vi "mapRotAngleByTiltXY.vi"(8 "error in (no error)":errorcluster, 9 "Tilt Angle (degree)":cluster{"Tile X":dbl, "Tilt Y":dbl}, 10 "Rotation Angle in Deg":dbl, 11 "CamRot in":refnum<class "CamRot.lvclass">) -> (0 "error out":errorcluster, 2 "Mapped Rotation Angle in Deg":dbl, 3 "CamRot out":refnum<class "CamRot.lvclass">)   [LabVIEW 2016, in "OfcFunc.lvlib" / "CamRot.lvclass"]
doc: "Map the rotation angle by tilt x, y axis. The input rotation angle (theta') is defined on x', y'-plane, which is tilted from x, y-plane. The output rotation angle (theta) is defined on x, y-plane. The tilt angles in inputs are defined as tilt x'-x and tilt y'-y."
uses:
  CamRot.lvclass
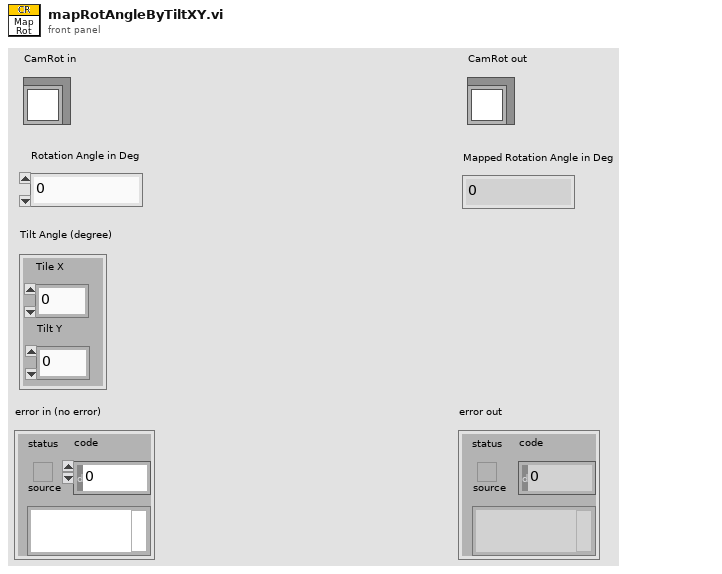
[diagram p1: front panel]
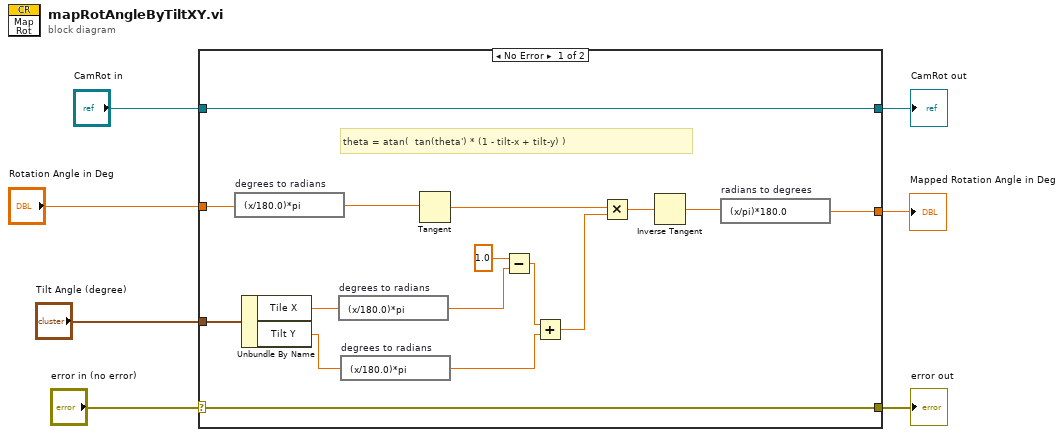
[diagram p0: block diagram]
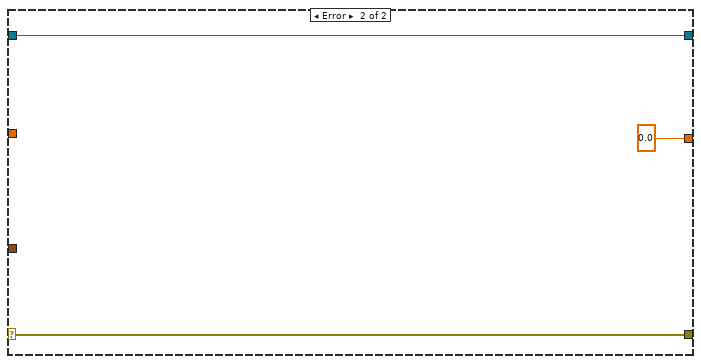
[diagram p2: hidden frame]
diagram:
  n1 = case shown="No Error" "error in (no error)" {
    selector: "error in (no error)" -> [w22 w26]
    tunnel: [w22 w26] -> w6
    tunnel: [w23 w25] -> w4
    tunnel: "CamRot in" -> [w23 w25]
    tunnel: "Rotation Angle in Deg" -> [w21 _]
    tunnel: "Tilt Angle (degree)" -> [w20 _]
    tunnel: [w17 0.0] -> w1
    frame No Error {
      # "theta = atan(  tan(theta') * (1 - tilt-x + tilt-y) )"
      n2 = expression code="(x/180.0)*pi" "degrees to radians"(w21) -> (w11:dbl)
      n3 = Unbundle By Name(w20) -> ("Tile X"=w19:dbl, "Tilt Y"=w18:dbl)
      n4 = expression code="(x/180.0)*pi" "degrees to radians"(w19) -> (w15:dbl)
      n5 = expression code="(x/180.0)*pi" "degrees to radians"(w18) -> (w13:dbl)
      n6 = Tangent(1:w11) -> (0:w10:dbl)
      n7 = Subtract(x=1.0, y=w15) -> (x-y=w14:dbl)
      n8 = Add(x=w14, y=w13) -> (x+y=w12:dbl)
      n9 = Multiply(x=w10, y=w12) -> (x*y=w9:dbl)
      n10 = Inverse Tangent(1:w9) -> (0:w8:dbl)
      n11 = expression code="(x/pi)*180.0" "radians to degrees"(w8) -> (w17:dbl)
    }
    frame Error {
    }
  }
  "error out" <- w6
  "CamRot out" <- w4
  "Mapped Rotation Angle in Deg" <- w1
